vi "runSingle.vi"(8 "error in (no error)":errorcluster, 11 "HWController in":refnum<class "HWController.lvclass">) -> (0 "error out":errorcluster, 1 "devicesConfigured":string[](array[string]), 2 "Stopped":bool, 3 "HWController out":refnum<class "HWController.lvclass">)   [LabVIEW 2011, in "Hardware.lvlib" / "HWControllers.lvlib" / "HWController.lvclass"]
uses:
  HWController.lvclass
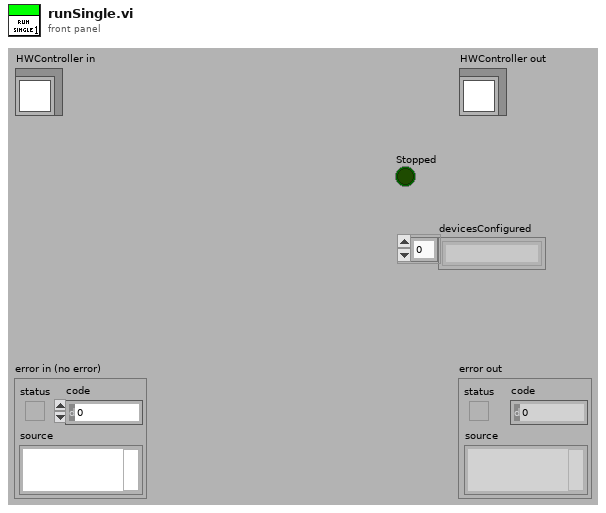
[diagram p1: front panel]
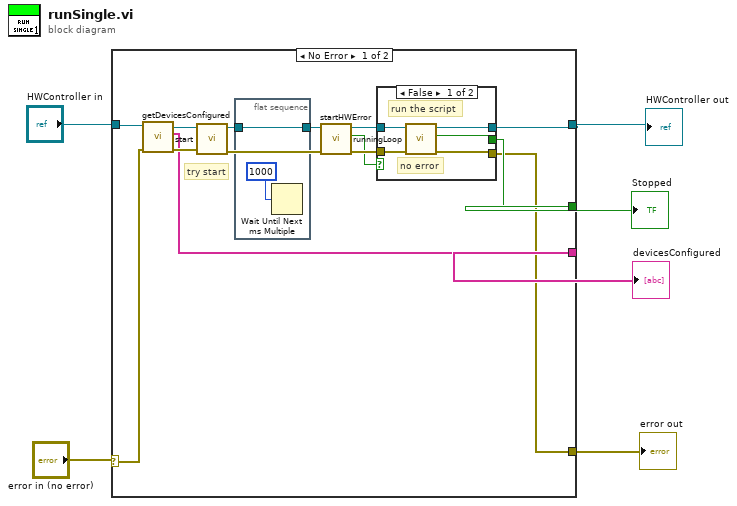
[diagram p0: block diagram]
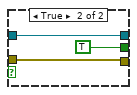
[diagram p2: hidden frame]
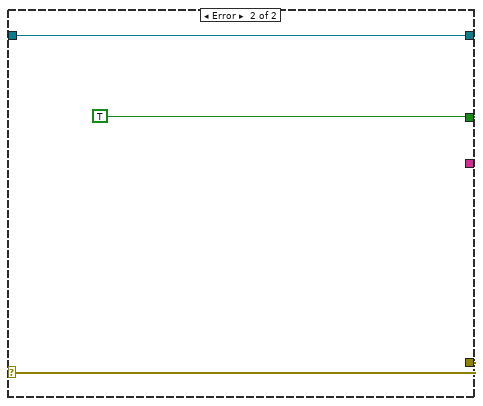
[diagram p3: hidden frame]
diagram:
  n1 = case shown="No Error" "error in (no error)" {
    selector: "error in (no error)" -> [w16 w33]
    tunnel: [w18 w33] -> w5
    tunnel: [w19 w32] -> w3
    tunnel: "HWController in" -> [w17 w32]
    tunnel: [w20 TRUE] -> w2
    tunnel: [w13 _] -> w1
    frame No Error {
      # "try start"
      n2 = call "getDevicesConfigured.vi"("error in (no error)"=w16, "HWController.lvclass in"=w17) -> ("error out"=w15:errorcluster, "devicesConfigured"=w13:string[], "HWController.lvclass out"=w14:refnum<class "HWController.lvclass">)  [unwired: 7 in]
      n3 = call-dynamic "start.vi"("error in (no error)"=w15, "HWController in"=w14) -> ("error out"=w12:errorcluster, "HWController out"=w7:refnum<class "HWController.lvclass">)  [unwired: 7 in, 1 out]
      n4 = flat-sequence {
        tunnel: [w22] -> w8
        tunnel: w7 -> [w22]
        frame #0 {
          n5 = Wait Until Next ms Multiple(millisecond multiple=1000) -> ()  [unwired: 1 out]
        }
      }
      n6 = call-dynamic "startHWError.vi"("error in (no error)"=w12, "HWController in"=w8) -> ("error out"=w10:errorcluster, "error"=w9:bool, "HWController out"=w11:refnum<class "HWController.lvclass">)  [unwired: 7 in]
      n7 = case shown="False" w9 {
        tunnel: [w27 TRUE] -> w20
        tunnel: [w26 w30] -> w19
        tunnel: [w25 w29] -> w18
        tunnel: w11 -> [w24 w30]
        tunnel: w10 -> [w23 w29]
        frame False {
          # "no error"
          # "run the script"
          n8 = call "runningLoop.vi"("error in (no error)"=w23, "HWController in"=w24) -> ("error out"=w25:errorcluster, "userStoped"=w27:bool, "HWController out"=w26:refnum<class "HWController.lvclass">)  [unwired: 7 in]
        }
        frame True {
        }
      }
    }
    frame Error {
    }
  }
  "error out" <- w5
  "HWController out" <- w3
  "Stopped" <- w2
  "devicesConfigured" <- w1
